vi "数组输入通道.vi"() -> ()   [LabVIEW 2023]
panel:
  out "内循环次数":i32
  out "外循环次数":i32
  out "循环数":i32
  in  "c":string[](array[string])
  in  "b":string[](array[string])
  in  "a":string[](array[string])
  out "输出2":string[][](array[string])
  out "输出":string
  in  "Array 2":string[][](array[string])
  out "concatenated string":string
  out "element":string
  out "array size(s)":i32
  in  "Array":string[](array[string])
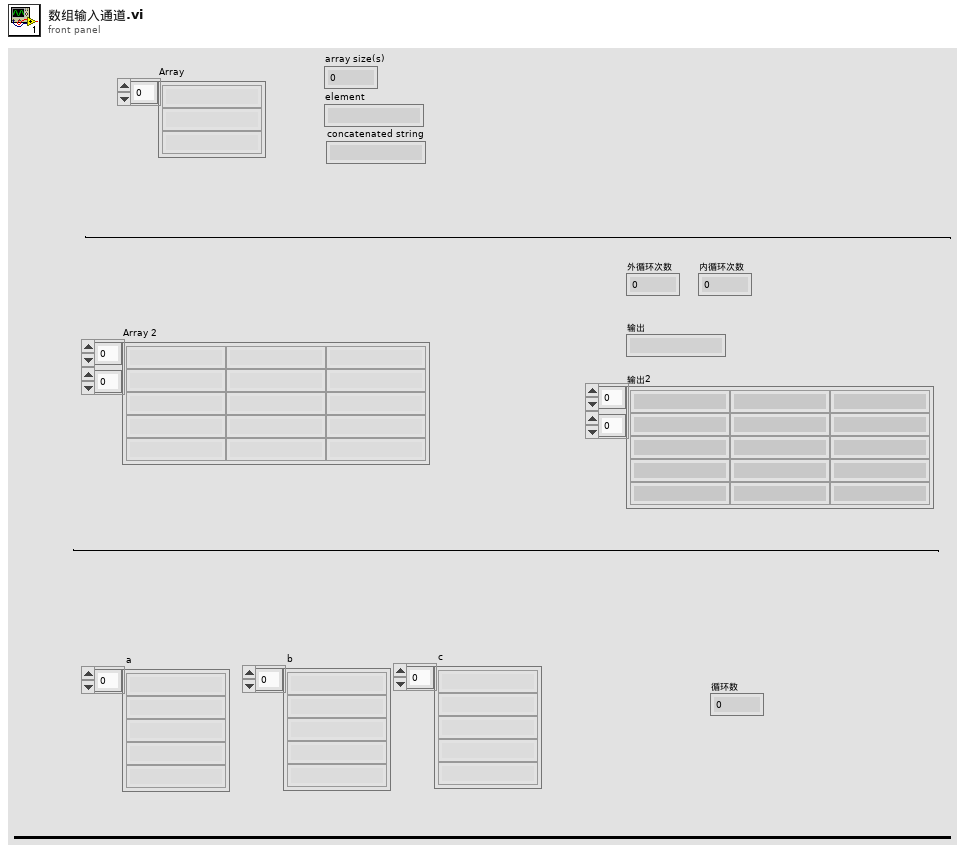
[diagram p1: front panel]
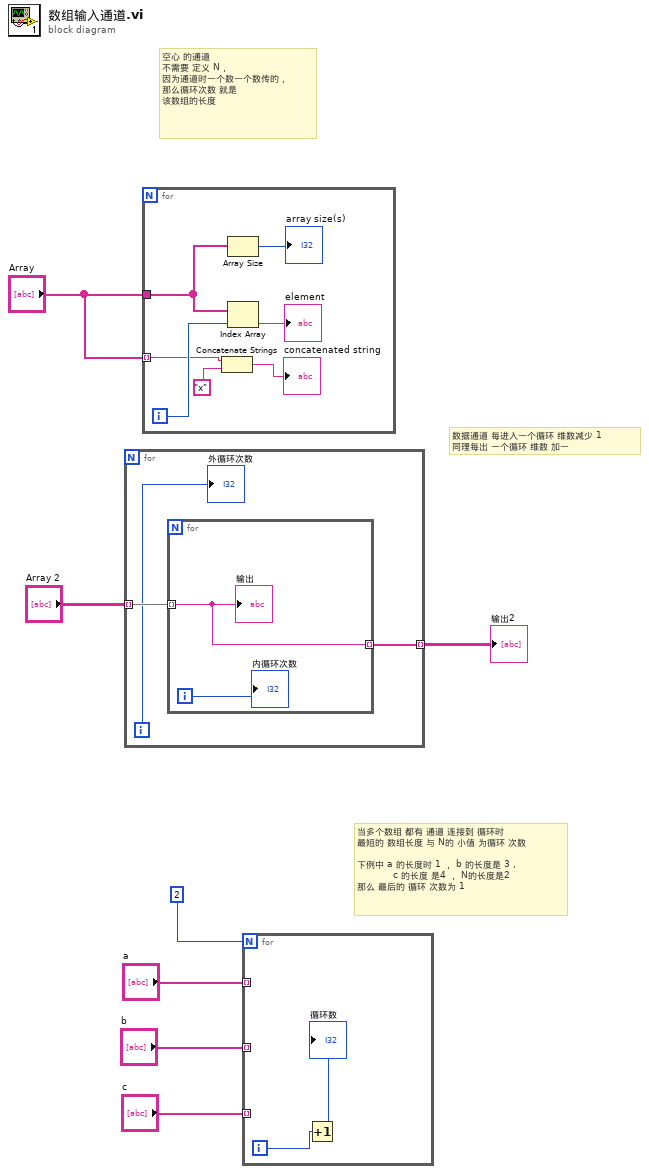
[diagram p0: block diagram]
diagram:
  # "当多个数组 都有 通道 连接到 循环时\n最短的 数组长度 与 N的 小值 为循环 次数\n\n下例中 a 的长度时 1 ， b 的长度是 3 , \n            c 的长度 是4 ， N的长度是2 \n那么 最后的 循环 次数为 1"
  # "数据通道 每进入一个循环 维数减少 1 \n同理每出 一个循环 维数 加一"
  # "空心 的通道\n不需要 定义 N， 因为通道时一个数一个数传的， 那么循环次数 就是\n该数组的长度"
  n1 = for {
    tunnel: "Array 2" -> [w10] mode=indexing
    tunnel: [w9] -> w5 mode=indexing
    i -> [w8]
    n2 = for {
      tunnel: w10 -> [w12] mode=indexing
      tunnel: [w12] -> w9 mode=indexing
      i -> [w11]
      "输出" <- w12
      "内循环次数" <- w11
    }
    "外循环次数" <- w8
  }
  "输出2" <- w5
  n3 = for {
    tunnel: "Array" -> [w18]
    tunnel: "Array" -> [w15] mode=indexing
    i -> [w17]
    n4 = Concatenate Strings(w15, "x" ("string")) -> (→"concatenated string":string)
    n5 = Array Size(array=w18) -> (size(s)=→"array size(s)":i32)
    n6 = Index Array(array=w18, index=w17) -> (element=→"element":string)
  }
  n7 = for {
    N: 2 -> [_]
    tunnel: "a" -> [_] mode=indexing
    tunnel: "b" -> [_] mode=indexing
    tunnel: "c" -> [_] mode=indexing
    i -> [w21]
    n8 = Increment(x=w21) -> (x+1=→"循环数":i32)
  }
